vi "PH_Tektronix_7000.Evt Call Set Channel Configuration.vi"(0 "i ref in":refnum<vi>, 1 "Instance":string="N/A", 2 "Channel":u16(ring) items=["Channel 1", "Channel 2", "Channel 3", "Channel 4", "Math 1", "Math 2", "Math 3", "Math 4", "Reference 1", "Reference 2", "Reference 3", "Reference 4"], 3 "Channel Configuration":T1={"Enable Channel"=FALSE, "Bandwidth"=0, "Input Impedance"=0, "Vertical Coupling"=0, "Probe Attenuation"=1.0, "Range [V/div]"=1.0, "Position [div]"=10.0, "Bandwidth raw"=""} {"Vertical Coupling" items=["AC", "DC", "Ground"]; "Input Impedance" items=["1M", "50"]; "Bandwidth" items=["FULL", "500 MHz", "250 MHz", "150 MHz", "20 MHz"]}, 5 "error in (no error)":errorcluster) -> (14 "i ref out":refnum<vi>, 19 "error out":errorcluster)   [LabVIEW 2014, in "PH_Tektronix_7000.lvlib"]
doc: "This VI calls sets a simple call."
uses:
  PH_Tektronix_7000.lvlib
  PH_Tektronix_7000.Channel Config.ctl
  CS_Core/CSSystem/CoreLib/CoreLib.short 2 byte array.vi
  CS_Core/CSSystem/CoreLib/CoreLib.double 2 byte array.vi
  CS_Core/CSSystem/CoreLib/CoreLib.lvlib
  CS_Core/BaseProcess/BaseProcess.lvlib
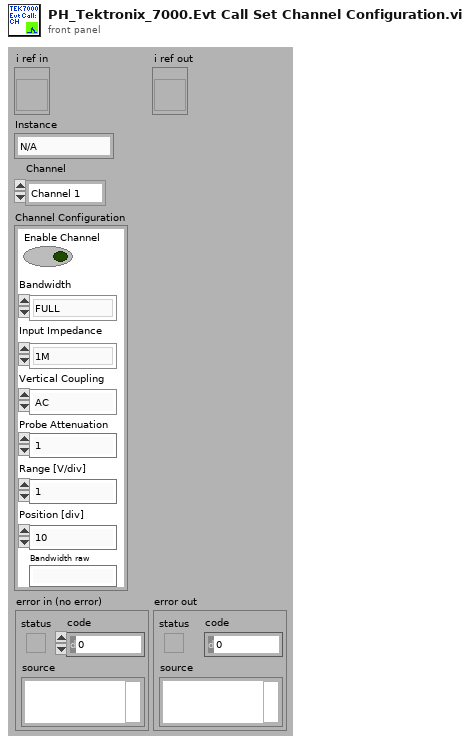
[diagram p1: front panel]
types:
  T1 = typedef "PH_Tektronix_7000.lvlib/PH_Tektronix_7000.Channel Config.ctl" = cluster{"Enable Channel":bool, "Bandwidth":u16, "Input Impedance":u16, "Vertical Coupling":u16, "Probe Attenuation":dbl, "Range [V/div]":dbl, "Position [div]":dbl, "Bandwidth raw":string}
  T2 = typedef "CoreDefs.rawDataType.ctl" = i8[]
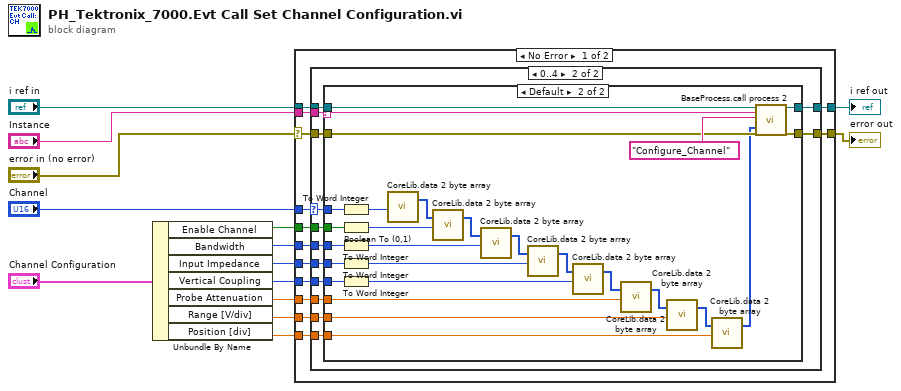
[diagram p0: block diagram]
diagram:
  n1 = Unbundle By Name("Channel Configuration") -> ("Enable Channel"=w8:bool, "Bandwidth"=w7:u16, "Input Impedance"=w6:u16, "Vertical Coupling"=w5:u16, "Probe Attenuation"=w4:dbl, "Range [V/div]"=w3:dbl, "Position [div]"=w2:dbl)
  n2 = case shown="No Error" "error in (no error)" {
    selector: "error in (no error)" -> [w23 w72]
    tunnel: [w27 w73] -> w14
    tunnel: [w26 w72] -> w13
    tunnel: "i ref in" -> [w25 w73]
    tunnel: "Channel" -> [w22 _]
    tunnel: "Instance" -> [w24 _]
    tunnel: w8 -> [w21 _]
    tunnel: w7 -> [w20 _]
    tunnel: w6 -> [w19 _]
    tunnel: w5 -> [w18 _]
    tunnel: w4 -> [w17 _]
    tunnel: w3 -> [w16 _]
    tunnel: w2 -> [w15 _]
    frame No Error {
      n3 = case shown="0..4" w22 {
        selector: w22 -> [_ w37]
        tunnel: [w29 w42] -> w27
        tunnel: [w28 w41] -> w26
        tunnel: w25 -> [w29 w40]
        tunnel: w24 -> [_ w39]
        tunnel: w23 -> [w28 w38]
        tunnel: w21 -> [_ w36]
        tunnel: w20 -> [_ w35]
        tunnel: w19 -> [_ w34]
        tunnel: w18 -> [_ w33]
        tunnel: w17 -> [_ w32]
        tunnel: w16 -> [_ w31]
        tunnel: w15 -> [_ w30]
        frame Default {
        }
        frame 0..4 {
          n4 = case shown="Default" w39 {
            selector: w39 -> [_ w66]
            tunnel: [w43 w70] -> w42
            tunnel: [w44 w69] -> w41
            tunnel: w40 -> [w43 w68]
            tunnel: w38 -> [w44 w67]
            tunnel: w37 -> [_ w65]
            tunnel: w36 -> [_ w64]
            tunnel: w35 -> [_ w62]
            tunnel: w34 -> [_ w57]
            tunnel: w33 -> [_ w56]
            tunnel: w32 -> [_ w54]
            tunnel: w31 -> [_ w51]
            tunnel: w30 -> [_ w50]
            frame "N/A" {
            }
            frame Default {
              n5 = To Word Integer(number=w65) -> (16bit integer=w45:i16)
              n6 = Boolean To (0,1)(Boolean=w64) -> (0, 1=w46:i16)
              n7 = To Word Integer(number=w62) -> (16bit integer=w47:i16)
              n8 = To Word Integer(number=w57) -> (16bit integer=w48:i16)
              n9 = To Word Integer(number=w56) -> (16bit integer=w55:i16)
              n10 = call-poly "CoreLib.data 2 byte array.vi"("i16"=w45) -> ("byteArray out"=w63:T2)  [unwired: 18 in]
              n11 = call-poly "CoreLib.data 2 byte array.vi"("byteArray"=w63, "i16"=w46) -> ("byteArray out"=w61:T2)  [unwired: 17 in]
              n12 = call-poly "CoreLib.data 2 byte array.vi"("byteArray"=w61, "i16"=w47) -> ("byteArray out"=w53:T2)  [unwired: 17 in]
              n13 = call-poly "CoreLib.data 2 byte array.vi"("byteArray"=w53, "i16"=w48) -> ("byteArray out"=w60:T2)  [unwired: 17 in]
              n14 = call-poly "CoreLib.data 2 byte array.vi"("byteArray"=w60, "i16"=w55) -> ("byteArray out"=w59:T2)  [unwired: 17 in]
              n15 = call-poly "CoreLib.data 2 byte array.vi"("byteArray"=w59, "f64"=w54) -> ("byteArray out"=w52:T2)  [unwired: 17 in]
              n16 = call-poly "CoreLib.data 2 byte array.vi"("byteArray"=w52, "f64"=w51) -> ("byteArray out"=w58:T2)  [unwired: 17 in]
              n17 = call-poly "CoreLib.data 2 byte array.vi"("byteArray"=w58, "f64"=w50) -> ("byteArray out"=w49:T2)  [unwired: 17 in]
              n18 = call "BaseProcess.call process 2.vi"("i ref in"=w68, "Object"=w66, "Selector"="Configure_Channel", "Data"=w49, "error in (no error)"=w67) -> ("i ref out"=w70:refnum<vi>, "error out"=w69:errorcluster)  [unwired: 13 in]
            }
          }
        }
      }
    }
    frame Error {
    }
  }
  "i ref out" <- w14
  "error out" <- w13
